vi "Log Message.vi"(8 "error in (no error)":errorcluster, 10 "Message":string, 11 "Logger in":refnum<class "Logger.lvclass">) -> (0 "error out":errorcluster, 3 "Logger out":refnum<class "Logger.lvclass">)   [LabVIEW 2020, in "GPack.lvlib" / "Logger.lvclass"]
uses:
  Logger.lvclass
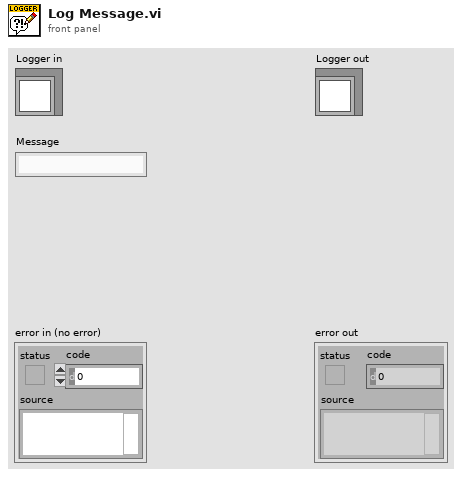
[diagram p1: front panel]
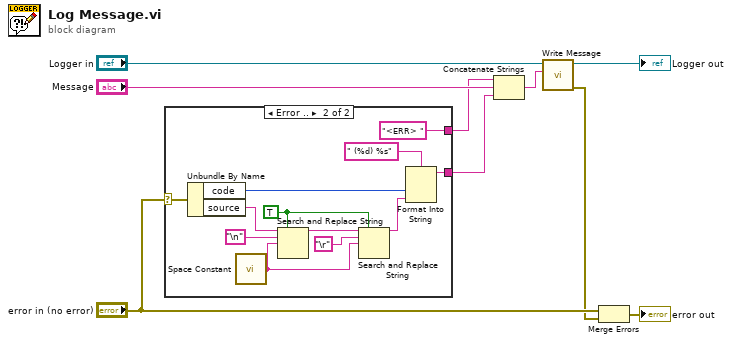
[diagram p0: block diagram]
diagram:
  n1 = case shown="Error .." "error in (no error)" {
    selector: "error in (no error)" -> [_ w21]
    tunnel: [_ w11] -> w6
    tunnel: [_ "<ERR> "] -> w1
    frame No Error {
    }
    frame Error {
      w15 = TRUE ("replace all? (F)")
      n2 = Unbundle By Name(w21) -> ("code"=w19:i32, "source"=w17:string)
      n3 = call <vilib>:"Space Constant.vi"() -> ("String"=w14:string)
      n4 = Search and Replace String(replace all?=w15, input string=w17, search string="\n", replace string=w14) -> (result string=w16:string)  [unwired: 4 in, 3 out]
      n5 = Search and Replace String(replace all?=w15, input string=w16, search string="\r", replace string=w14) -> (result string=w12:string)  [unwired: 4 in, 3 out]
      n6 = Format Into String(format string=" (%d) %s", w19, w12) -> (resulting string=w11:string)  [unwired: 2 in, 1 out]
    }
  }
  n7 = Concatenate Strings(w1, "Message", w6) -> (w4:string)
  n8 = call-dynamic "Write Message.vi"("Message"=w4, "Logger in"="Logger in") -> ("error out"=w2:errorcluster, "Logger out"=→"Logger out":refnum<class "Logger.lvclass">)  [unwired: 8 in]
  n9 = Merge Errors("error in (no error)", w2) -> (→"error out":errorcluster)
